vi "曲线鼠标悬停显示信息.vi"() -> ()   [LabVIEW 2013]
uses:
  <vilib>/Utility/miscctls.llb/LVPoint32TypeDef.ctl
panel:
  in  "曲线.可见":bool
  in  "活动曲线":u32
  out "Y":dbl
  out "X":dbl
  out "y":dbl
  out "x":dbl
  out "坐标":cluster{"数组":i32[], "数组":i32[]}
  out "x-y":dbl
  out "坐标对映射数组":T1[](array[typedef])
  out "XY图":cluster{dbl[], dbl[]}[](graph)
  in  "停止按钮":bool
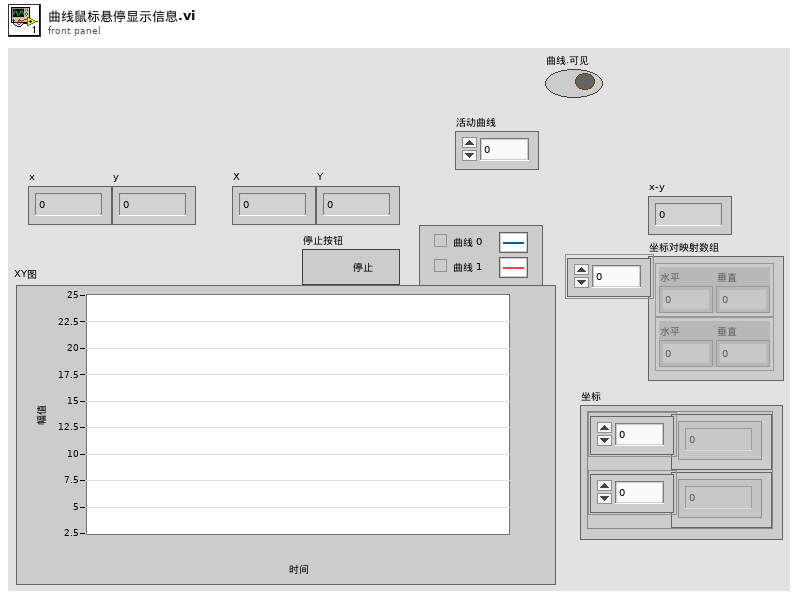
[diagram p1: front panel]
types:
  T1 = typedef "LVPoint32TypeDef.ctl" = cluster{"Horizontal":i32, "Vertical":i32}
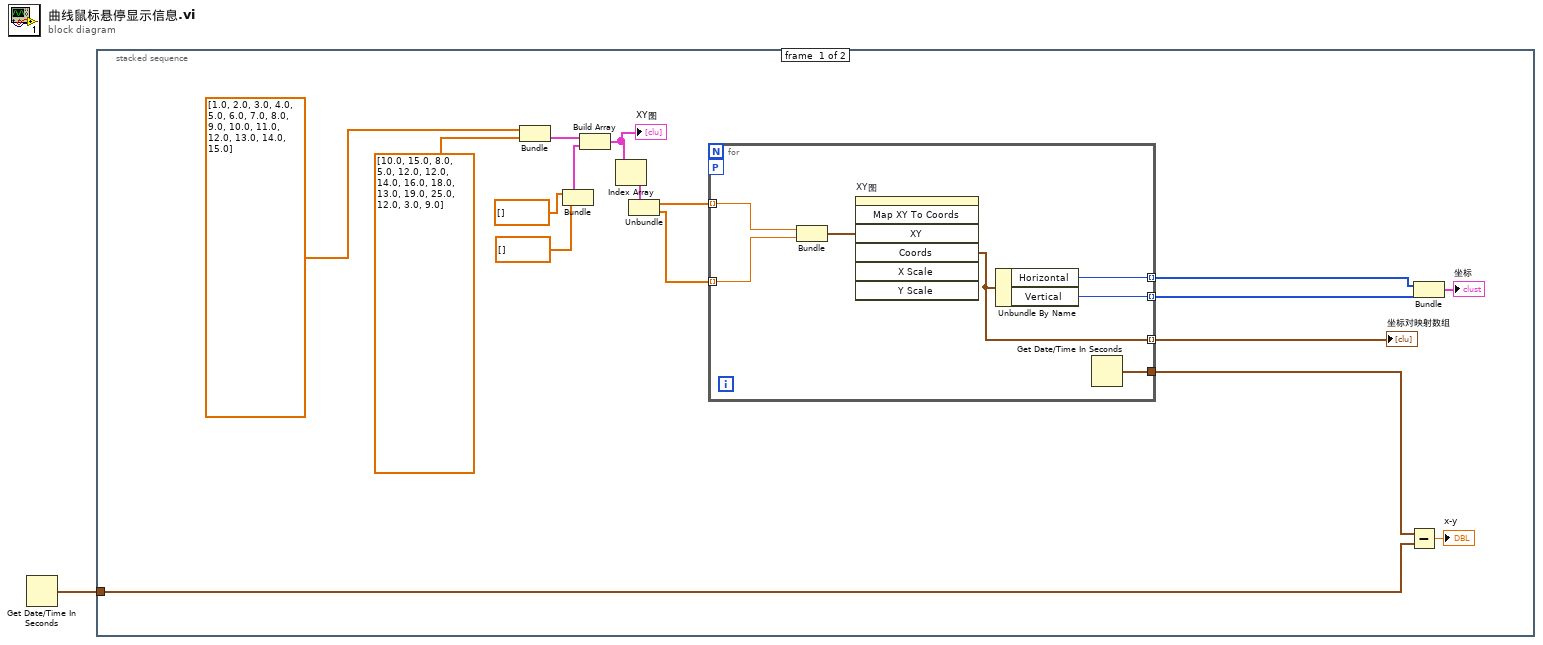
[diagram p0: block diagram]
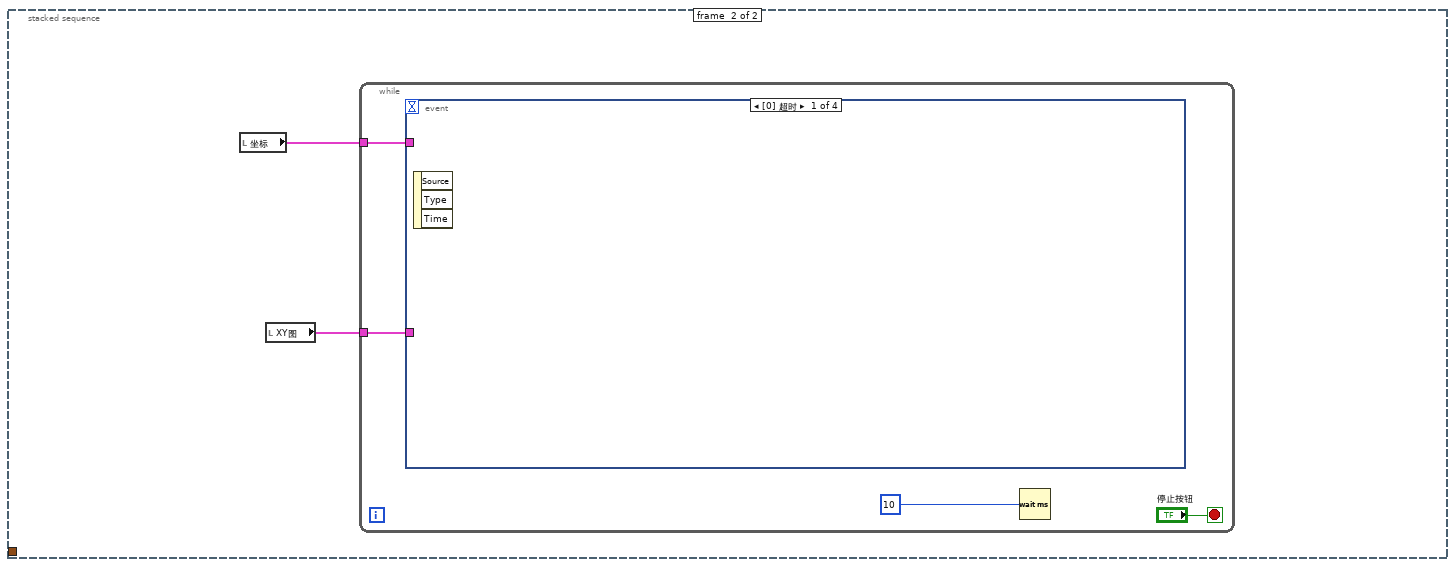
[diagram p2: hidden frame]
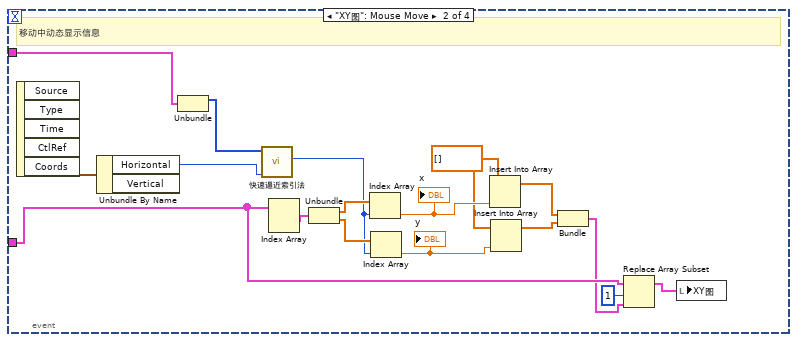
[diagram p3: hidden frame]
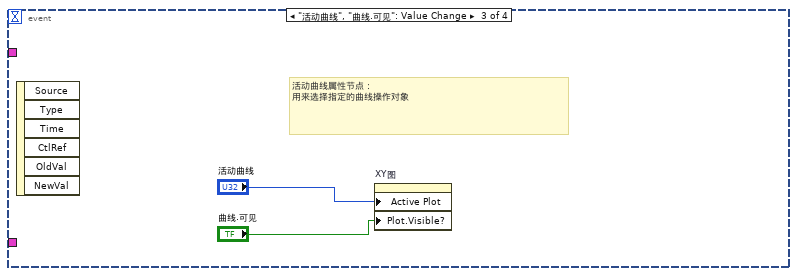
[diagram p4: hidden frame]
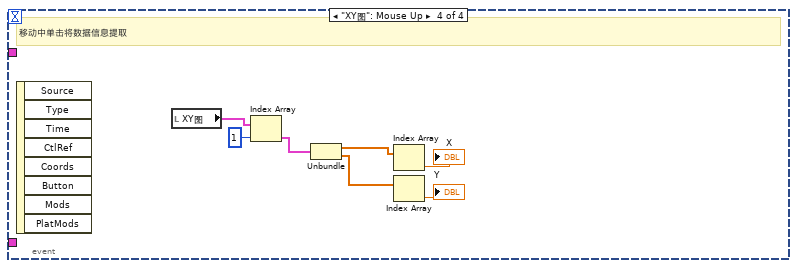
[diagram p5: hidden frame]
diagram:
  n1 = Get Date/Time In Seconds() -> (seconds since 1Jan1904=w1:timestamp)
  n2 = stacked-sequence {
    tunnel: w1 -> [w13 _]
    frame #0 {
      n3 = Bundle(dbl[] [1.0, 2.0, 3.0, 4.0, 5.0, 6.0, 7.0, 8.0, 9.0, 10.0, 11.0, 12.0, 13.0, 14.0, 15.0], dbl[] [10.0, 15.0, 8.0, 5.0, 12.0, 12.0, 14.0, 16.0, 18.0, 13.0, 19.0, 25.0, 12.0, 3.0, 9.0]) -> (w10:cluster{dbl[], dbl[]})  [unwired: 1 in]
      n4 = Bundle(dbl[] [], dbl[] []) -> (w8:cluster{dbl[], dbl[]})  [unwired: 1 in]
      n5 = Build Array(w10, w8) -> (w9:cluster{dbl[], dbl[]}[])
      "XY图" <- w9
      n6 = Index Array(array=w9) -> (element=w5:cluster{dbl[], dbl[]})  [unwired: 1 in]
      n7 = Unbundle(w5) -> (w16:dbl[], w15:dbl[])
      n8 = for {
        tunnel: w16 -> [w25] mode=indexing
        tunnel: w15 -> [w24] mode=indexing
        tunnel: [w21] -> w11 mode=indexing
        tunnel: [w22] -> w14
        workers-P: _ -> [_]
        tunnel: [w20] -> w4 mode=indexing
        tunnel: [w19] -> w3 mode=indexing
        n9 = Bundle(w25, w24) -> (w23:cluster{dbl, dbl})  [unwired: 1 in]
        n10 = invoke on="XY图" class="XYGraph (严格)" method="Map XY To Coords"("XY"=w23) -> ("Coords"=w21:T1)  [unwired: 6 in, 6 out]
        n11 = Unbundle By Name(w21) -> ("Horizontal"=w20:i32, "Vertical"=w19:i32)
        n12 = Get Date/Time In Seconds() -> (seconds since 1Jan1904=w22:timestamp)
      }
      "坐标对映射数组" <- w11
      n13 = Subtract(x=w14, y=w13) -> (x-y=→"x-y":dbl)
      n14 = Bundle(w4, w3) -> (→"坐标":cluster{i32[], i32[]})  [unwired: 1 in]
    }
    frame #1 {
      n15 = local read "坐标"() -> (w26:cluster{"数组":i32[], "数组":i32[]})
      n16 = local read "XY图"() -> (w27:cluster{dbl[], dbl[]}[])
      n17 = while {
        tunnel: w27 -> [w29]
        tunnel: w26 -> [w28]
        stop <- "停止按钮" stop-if-true
        n18 = event shown="[0] 超时" {
          selector: _ -> [_ _ _ _]
          dyn-events: _ -> [_ _ _ _]
          timeout: _ -> [_ _ _ _]
          tunnel: w29 -> [_ w34 _ _]
          tunnel: w28 -> [_ w46 _ _]
          event Timeout {
            n19 = event-data() -> ()  [unwired: 1 in, 3 out]
          }
          event "XY图": Mouse Move {
            w38 = dbl[] [] ("数组")
            # "移动中动态显示信息"
            n20 = event-data() -> ("Coords"=w48:T1)  [unwired: 1 in, 4 out]
            n21 = Unbundle By Name(w48) -> ("Horizontal"=w47:i32)  [unwired: 1 out]
            n22 = Unbundle(w46) -> ("数组"=w45:i32[])  [unwired: 1 out]
            n23 = call "快速逼近索引法.vi"("数值"=w47, "数组"=w45) -> ("最近索引"=w41:i32)  [unwired: 9 in]
            n24 = Index Array(array=w34) -> (element #1=w43:cluster{dbl[], dbl[]})  [unwired: 2 in, 1 out]
            n25 = Unbundle(w43) -> (w44:dbl[], w42:dbl[])
            n26 = Index Array(array=w44, index=w41) -> (element=w40:dbl)
            "x" <- w40
            n27 = Index Array(array=w42, index=w41) -> (element=w39:dbl)
            "y" <- w39
            n28 = Insert Into Array(array=w38, new element=w40) -> (w37:dbl[])  [unwired: 1 in]
            n29 = Insert Into Array(array=w38, new element=w39) -> (w36:dbl[])  [unwired: 1 in]
            n30 = Bundle("数组"=w37, "数组"=w36) -> (w33:cluster{"数组":dbl[], "数组":dbl[]})  [unwired: 1 in]
            n31 = Replace Array Subset(array=w34, new element=w33, index=1 ("索引")) -> (w32:cluster{dbl[], dbl[]}[])
            n32 = local write "XY图"(w32) -> ()
          }
          event "活动曲线", "曲线.可见": Value Change {
            # "活动曲线属性节点：\n用来选择指定的曲线操作对象"
            n33 = event-data() -> ()  [unwired: 1 in, 6 out]
            n34 = property on="XY图" class="XYGraph (严格)"("Active Plot"="活动曲线", "Plot.Visible?"="曲线.可见") -> ()  [unwired: 2 in, 2 out]
          }
          event "XY图": Mouse Up {
            # "移动中单击将数据信息提取"
            n35 = event-data() -> ()  [unwired: 1 in, 8 out]
            n36 = local read "XY图"() -> (w57:cluster{dbl[], dbl[]}[])
            n37 = Index Array(array=w57, index=1 ("索引")) -> (element=w55:cluster{dbl[], dbl[]})
            n38 = Unbundle(w55) -> (w54:dbl[], w53:dbl[])
            n39 = Index Array(array=w54) -> (element=→"X":dbl)  [unwired: 1 in]
            n40 = Index Array(array=w53) -> (element=→"Y":dbl)  [unwired: 1 in]
          }
        }
        n41 = Wait (ms)(milliseconds to wait=u32 10 ("等待时间（毫秒）")) -> ()  [unwired: 1 out]
      }
    }
  }
